vi "FPGA Target Approach RetractionA1.vi"() -> ()   [LabVIEW 2012]
uses:
  <vilib>/rvi/FXPMathLib/basic elements/FxpIntAccumulator/subVIs/nifxpmath_IntAccumulator_SimConfig.ctl
  <vilib>/rvi/eio/common/nirviEmuTemplateMethod_errors.vi
  <vilib>/rvi/interface/RandomDataEmulation/nirviRandomDataFPGAFIFO.vi
  <vilib>/rvi/interface/RandomDataEmulation/niFpgaRandomDataHandleErrors.vi
  <vilib>/rvi/Emulation/niFpgaSctlEmulationGetInTimedLoop.vi
  <vilib>/rvi/FXPMathLib/basic elements/FxpIntAccumulator/simVIs/DllFxpIntAccumulator_sub.vi
  <vilib>/rvi/Emulation/niFpgaSctlEmulationGlobalWrite.vi
  <vilib>/eio/EIONode/EIONode.xnode
  <vilib>/rvi/DataTransferAndStorage/Container/XNode/niFpgaContainer.xnode
  <vilib>/rvi/interface/RandomDataEmulation/nirviRandomDataFpgaReadWriteTemplate.vi
  <vilib>/rvi/Analysis/measure/butterworth/XNode/niFpgaButterworthFilter.xnode
  <vilib>/rvi/FXPMathLib/basic elements/FxpIntAccumulator/XNode/nifxpmath_IntAccumulator.xnode
panel:
  out "Test Case Number Indicator":i16
  in  "Fast Approach Speed":fxp<+,64,38>
  in  "Test Case Number":i16
  in  "Manual":bool
  in  "Approach":bool
  out "Summation":fxp<+/-,64,38>
  in  "Data Acquisition Rate":i16
  out "Ticks":i16
  out "HV/10":i16
  out "Tuning Fork Signal":fxp<+/-,24,17>
  in  "Fast Retraction Speed":fxp<+,64,38>
  out "FPGA Output Voltage":fxp<+/-,64,32>
  out "Z Fine Indicator":fxp<+/-,40,30>
  out "Counter Indicator":fxp<+/-,64,32>
  in  "Z Fine Output":fxp<+/-,40,30>
  in  "Counter Output":i32
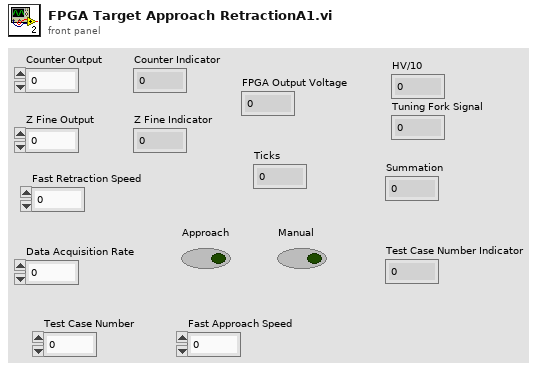
[diagram p1: front panel]
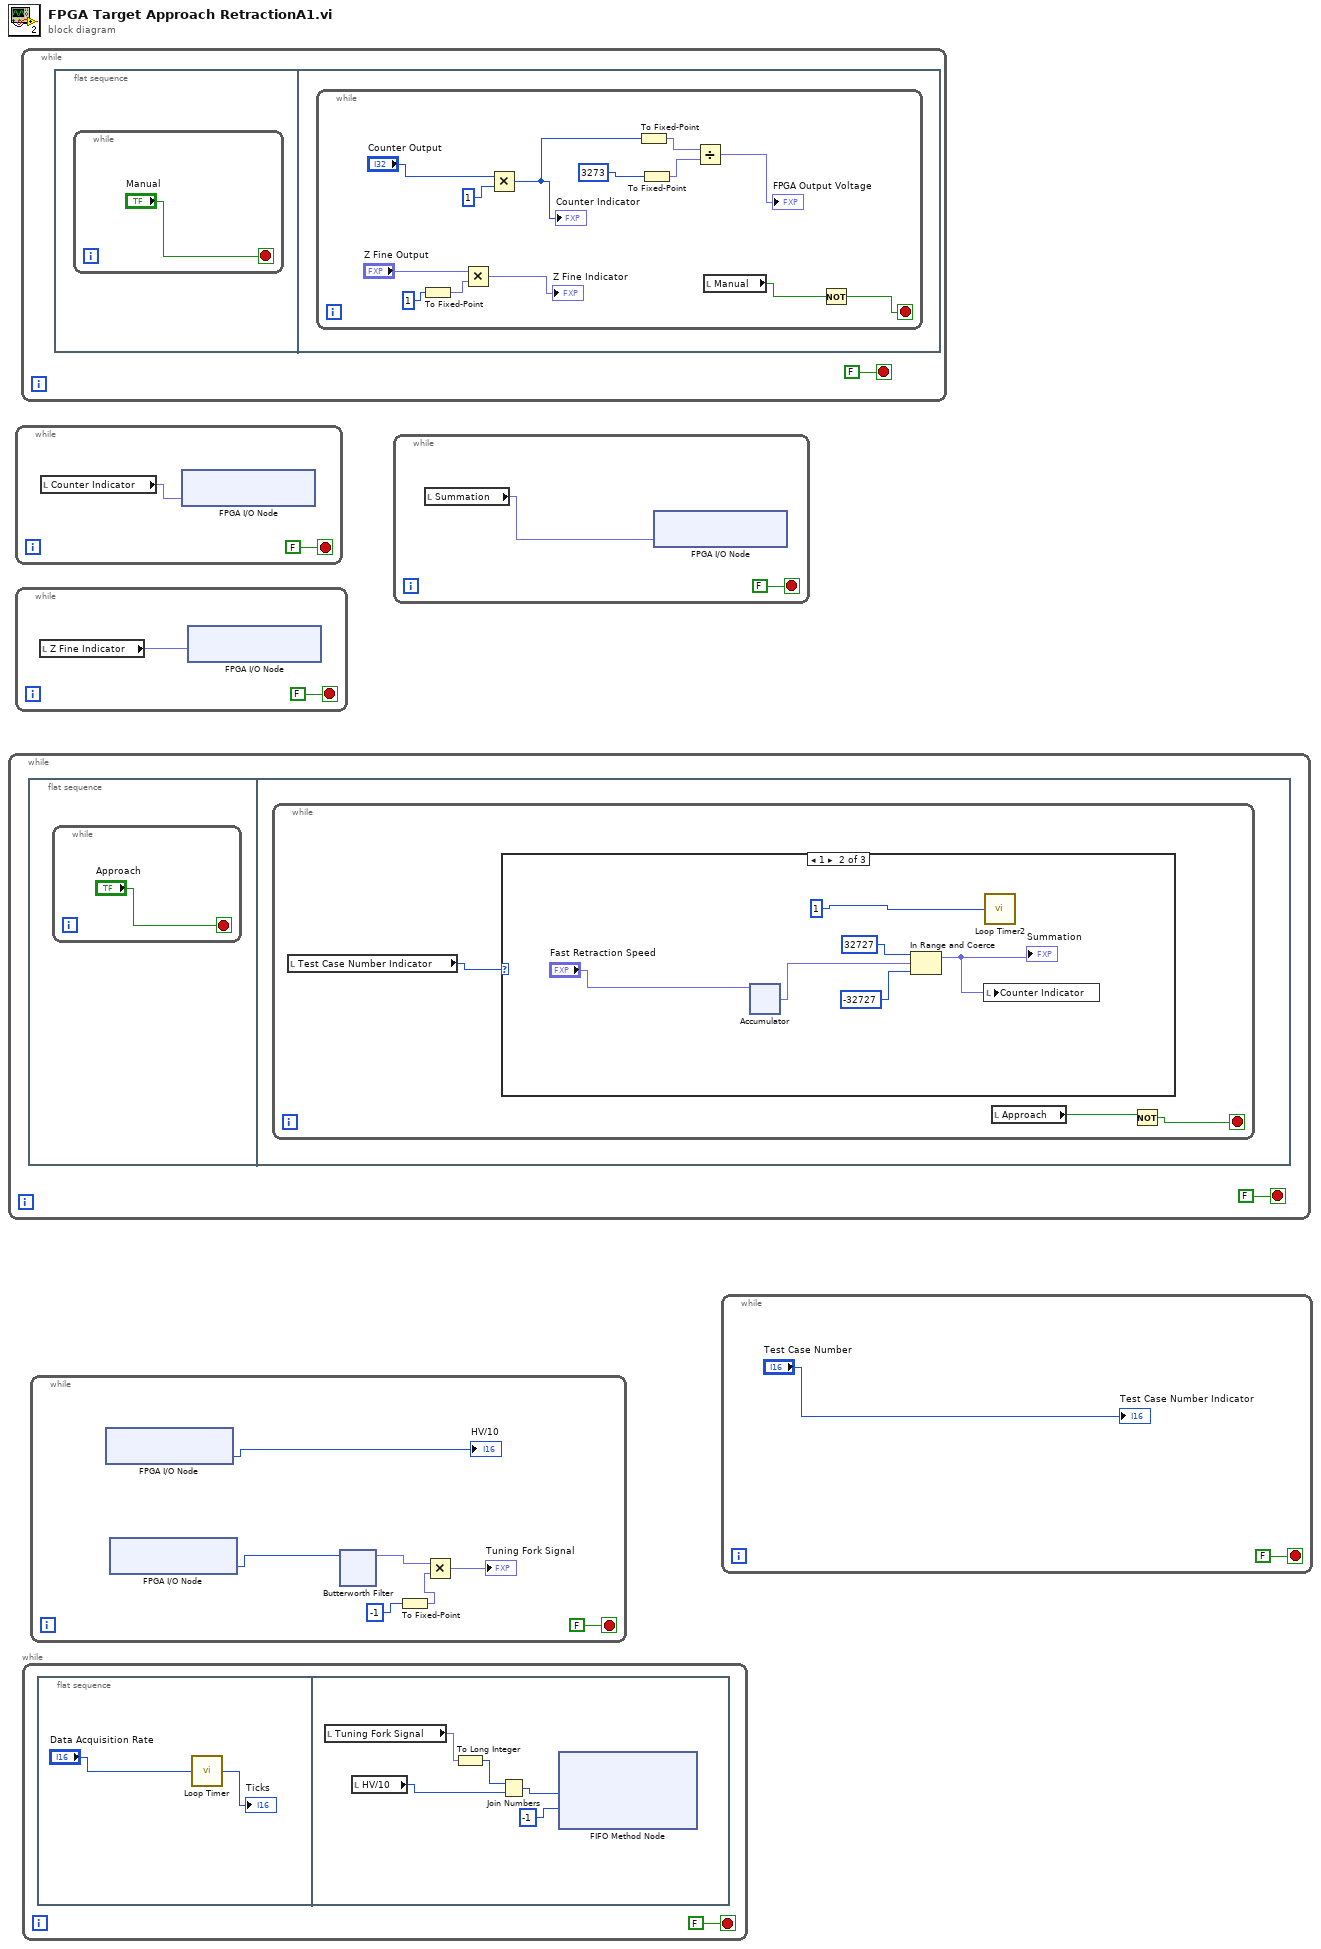
[diagram p0: block diagram]
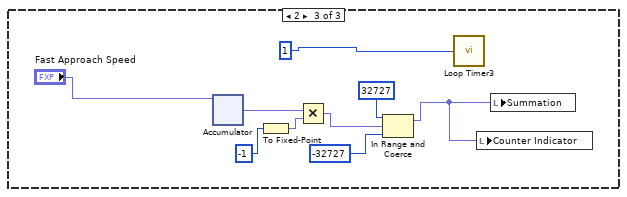
[diagram p3: hidden frame]
diagram:
  n1 = while {
    stop <- FALSE stop-if-true
    n2 = flat-sequence {
      frame #0 {
        n3 = while {
          stop <- "Approach" stop-if-true
        }
      }
      frame #1 {
        n4 = while {
          stop <- w4 stop-if-true
          n5 = local read "Test Case Number Indicator"() -> (w3:i16)
          n6 = case shown="1" w3 {
            frame 3, Default {
            }
            frame 1 {
              n7 = xnode "Accumulator"("x"="Fast Retraction Speed") -> ("s"=w9:fxp<+,64,38>)  [unwired: 4 in, 1 out]
              n8 = In Range and Coerce(upper limit=i16 32727, x=w9, lower limit=i16 -32727) -> (coerced(x)=w6:fxp<+/-,64,39>)  [unwired: 1 out]
              "Summation" <- w6
              n9 = local write "Counter Indicator"(w6) -> ()
              n10 = call "Loop Timer2"("Count(uSec)"=i16 1) -> ()  [unwired: 1 out]
            }
            frame 2 {
              n11 = xnode "Accumulator"("x"="Fast Approach Speed") -> ("s"=w39:fxp<+,64,38>)  [unwired: 4 in, 1 out]
              n12 = To Fixed-Point(number=i16 -1) -> (fixed-point=w41:fxp<+/-,16,16>)  [unwired: 1 in]
              n13 = Multiply(x=w39, y=w41) -> (x*y=w42:fxp<+/-,64,54>)
              n14 = In Range and Coerce(upper limit=i16 32727, x=w42, lower limit=i16 -32727) -> (coerced(x)=w43:fxp<+/-,64,54>)  [unwired: 1 out]
              n15 = call "Loop Timer3"("Count(uSec)"=i16 1) -> ()  [unwired: 1 out]
              n16 = local write "Counter Indicator"(w43) -> ()
              n17 = local write "Summation"(w43) -> ()
            }
          }
          n18 = local read "Approach"() -> (w5:bool)
          n19 = Not(x=w5) -> (.not. x?=w4:bool)
        }
      }
    }
  }
  n20 = while {
    stop <- FALSE stop-if-true
    n21 = local read "Counter Indicator"() -> (w75:fxp<+/-,64,32>)
    n22 = xnode "FPGA I/O Node"("Connector0/AO7"=w75) -> ()  [unwired: 1 in, 1 out]
  }
  n23 = while {
    stop <- FALSE stop-if-true
    n24 = local read "Z Fine Indicator"() -> (w77:fxp<+/-,40,30>)
    n25 = xnode "FPGA I/O Node"("Connector0/AO2"=w77) -> ()  [unwired: 1 in, 1 out]
  }
  n26 = while {
    stop <- FALSE stop-if-true
    n27 = flat-sequence {
      frame #0 {
        n28 = while {
          stop <- "Manual" stop-if-true
        }
      }
      frame #1 {
        n29 = while {
          stop <- w81 stop-if-true
          n30 = To Fixed-Point(number=1) -> (fixed-point=w89:fxp<+/-,32,32>)  [unwired: 1 in]
          n31 = Multiply(x="Z Fine Output", y=w89) -> (x*y=→"Z Fine Indicator":fxp<+/-,64,62>)
          n32 = Multiply(x="Counter Output", y=1) -> (x*y=w87:i32)
          "Counter Indicator" <- w87
          n33 = To Fixed-Point(number=w87) -> (fixed-point=w86:fxp<+/-,32,32>)  [unwired: 1 in]
          n34 = To Fixed-Point(number=3273) -> (fixed-point=w85:fxp<+/-,32,32>)  [unwired: 1 in]
          n35 = Divide(x=w86, y=w85) -> (x/y=→"FPGA Output Voltage":fxp<+/-,64,33>)
          n36 = local read "Manual"() -> (w82:bool)
          n37 = Not(x=w82) -> (.not. x?=w81:bool)
        }
      }
    }
  }
  n38 = while {
    stop <- FALSE stop-if-true
    n39 = flat-sequence {
      frame #0 {
        n40 = call "Loop Timer"("Count(uSec)"="Data Acquisition Rate") -> ("Tick Count(uSec)"=→"Ticks":u32)
      }
      frame #1 {
        n41 = local read "Tuning Fork Signal"() -> (w101:fxp<+/-,24,17>)
        n42 = local read "HV/10"() -> (w100:i16)
        n43 = To Long Integer(number=w101) -> (32bit integer=w99:i32)
        n44 = Join Numbers(hi=w99, lo=w100) -> ((hi.lo)=w98:u64)
        n45 = xnode ("FIFO Method Node")("Element"=w98, "Timeout"=i16 -1) -> ()  [unwired: 1 in, 2 out]
      }
    }
  }
  n46 = while {
    stop <- FALSE stop-if-true
    n47 = xnode "FPGA I/O Node"() -> ("Connector0/AI6"=→"HV/10":i16)  [unwired: 1 in, 1 out]
    n48 = xnode "FPGA I/O Node"() -> ("Connector0/AI7"=w107:i16)  [unwired: 1 in, 1 out]
    n49 = xnode "Butterworth Filter"("input data"=w107) -> ("output data"=w103:fxp<+/-,20,20>)  [unwired: 2 in]
    n50 = To Fixed-Point(number=i16 -1) -> (fixed-point=w104:fxp<+/-,16,16>)  [unwired: 1 in]
    n51 = Multiply(x=w103, y=w104) -> (x*y=→"Tuning Fork Signal":fxp<+/-,36,36>)
  }
  n52 = while {
    stop <- FALSE stop-if-true
    n53 = local read "Summation"() -> (w117:fxp<+/-,64,38>)
    n54 = xnode "FPGA I/O Node"("Connector0/AO4"=w117) -> ()  [unwired: 1 in, 1 out]
  }
  n55 = while {
    stop <- FALSE stop-if-true
    "Test Case Number Indicator" <- "Test Case Number"
  }
